vi "Connect Port.vi"(6 "timeout ms":i32=5000, 8 "error in":errorcluster, 9 "remote port":u16, 10 "address":string, 11 "NetStream in":refnum<class "NetStream.lvclass">) -> (0 "error out":errorcluster, 2 "Remote connected?":bool, 3 "NetStream out":refnum<class "NetStream.lvclass">)   [LabVIEW 2022 SP3, in "hse-network.lvlib" / "NetStream.lvclass"]
doc: "____\nHAMPEL SOFTWARE ENGINEERING v3.8.0 (2023-12-18 14:41)"
uses:
  NetStream.lvclass
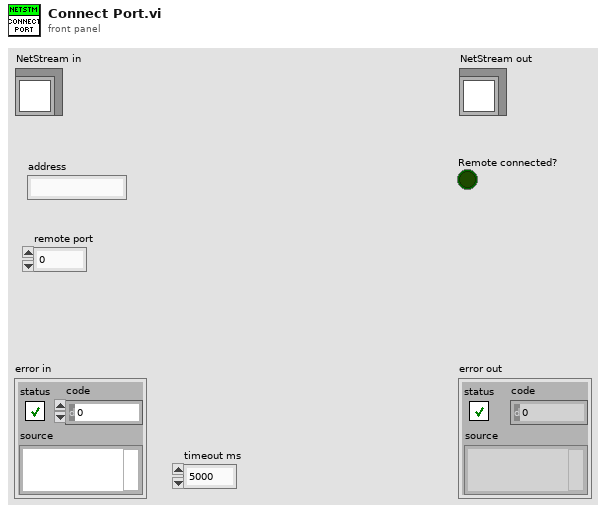
[diagram p1: front panel]
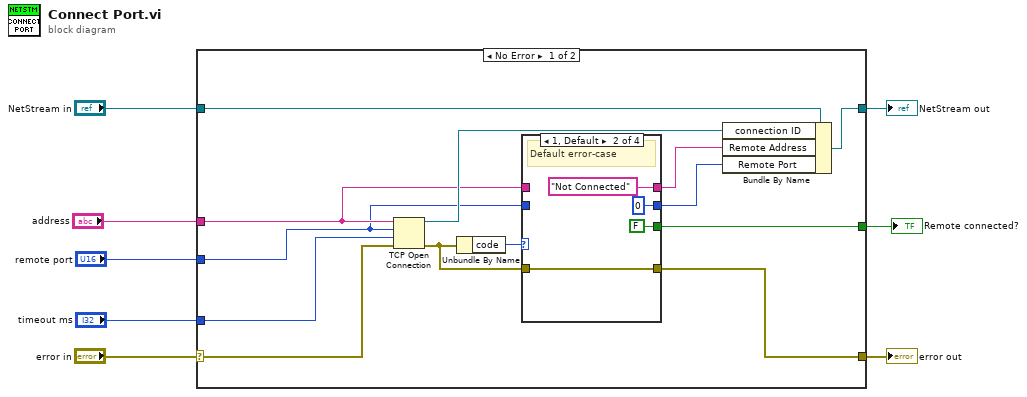
[diagram p0: block diagram]
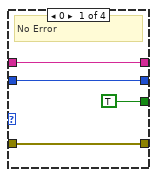
[diagram p2: hidden frame]
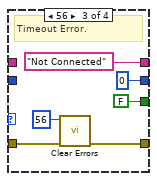
[diagram p3: hidden frame]
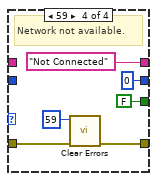
[diagram p4: hidden frame]
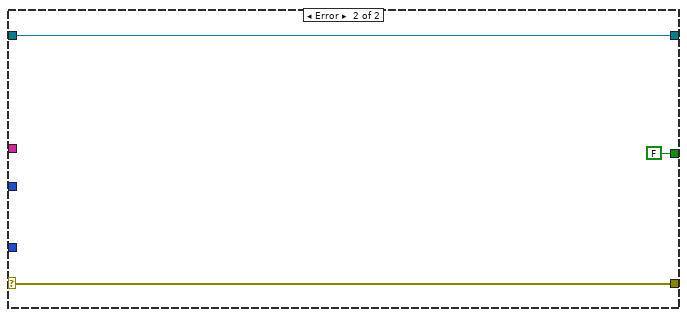
[diagram p5: hidden frame]
diagram:
  n1 = case shown="No Error" "error in" {
    selector: "error in" -> [w21 w44]
    tunnel: [w13 w44] -> w7
    tunnel: [w19 w43] -> w5
    tunnel: "NetStream in" -> [w17 w43]
    tunnel: "address" -> [w12 _]
    tunnel: "remote port" -> [w11 _]
    tunnel: "timeout ms" -> [w20 _]
    tunnel: [w14 FALSE] -> w1
    frame No Error {
      n2 = TCP Open Connection(address=w12, remote port or service name=w11, timeout ms (60000)=w20, error in (no error)=w21) -> (connection ID=w18:refnum<k5>, error out=w15:errorcluster)  [unwired: 1 in]
      n3 = Unbundle By Name(w15) -> ("code"=w16:i32)
      n4 = case shown="1, Default" w16 {
        tunnel: w15 -> [w25 w26 w34 w41]
        tunnel: [TRUE FALSE FALSE FALSE] -> w14
        tunnel: [w25 w26 w32 w40] -> w13
        tunnel: w12 -> [w23 _ _ _]
        tunnel: w11 -> [w22 _ _ _]
        tunnel: [w22 u16 0 ("remote port") u16 0 ("remote port") u16 0 ("remote port")] -> w10
        tunnel: [w23 "Not Connected" ("str_Remote_IP") "Not Connected" ("str_Remote_IP") "Not Connected" ("str_Remote_IP")] -> w9
        frame 0 {
          # "No Error"
        }
        frame 1, Default {
          # "Default error-case"
        }
        frame 56 {
          # "Timeout Error."
          n5 = call <vilib>:"Clear Errors.vi"("error in (no error)"=w34, "specific error code to clear (0: all)"=56) -> ("error out"=w32:errorcluster)  [unwired: 4 in, 1 out]
        }
        frame 59 {
          # "Network not available."
          n6 = call <vilib>:"Clear Errors.vi"("error in (no error)"=w41, "specific error code to clear (0: all)"=59) -> ("error out"=w40:errorcluster)  [unwired: 4 in, 1 out]
        }
      }
      n7 = Bundle By Name(cluster=w17, "connection ID"=w18, "Remote Address"=w9, "Remote Port"=w10) -> (w19:refnum<class "NetStream.lvclass">)
    }
    frame Error {
    }
  }
  "error out" <- w7
  "NetStream out" <- w5
  "Remote connected?" <- w1
